vi "BallChaseAuton.vi"(9 "milliseconds to fire":u32=750) -> ()   [LabVIEW 2013]
uses:
  Auton sequence.ctl
  Events.vi
  TwoBallAuton.ctl
panel:
  out "State":T1=enum."GetBall"
  out "GrabCount":i32
  out "Direction saw last":dbl
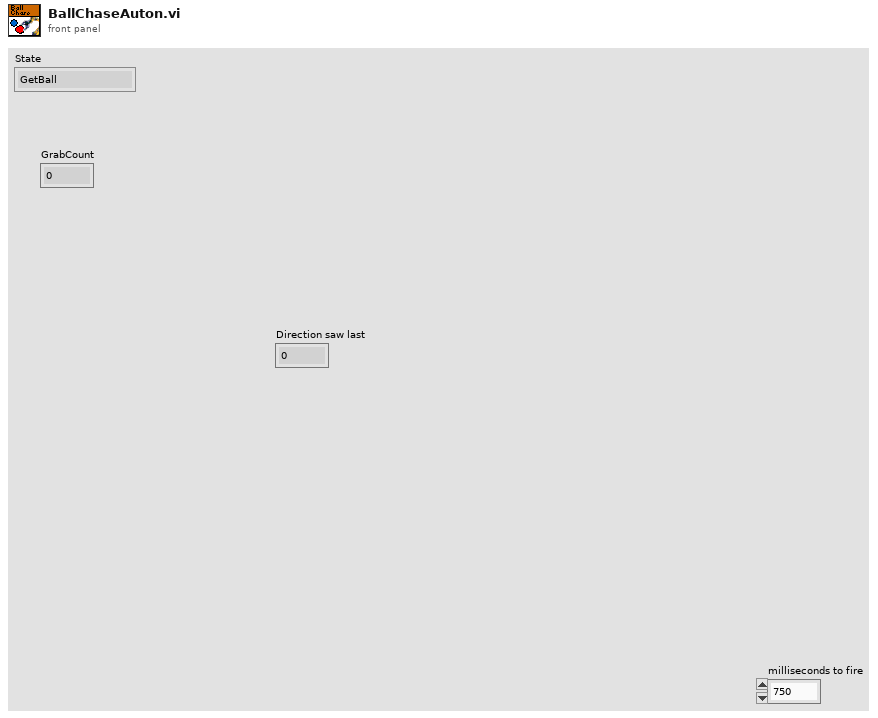
[diagram p1: front panel]
types:
  T1 = typedef "TwoBallAuton.ctl" = enum16{"Start", "LineUp", "Fire", "Reload", "GetBall", "Finish"}
  T2 = typedef "Auton sequence.ctl" = enum16{"Done", "move", "Shoot Ball 2", "Aquire target", "Ball chase", "Turn 90 ", "Shoot Ball 1"}
  T3 = typedef "WPI_SolenoidValue.ctl" = enum16{"Off", "On", "Forward", "Reverse"}
  T4 = cluster{"Ultrasonic Distance (In)":dbl, "Gyro":dbl, "TopAquisition sensor":bool, "Encoder distance":dbl, "Encoder rate":dbl, "Encoder direction":bool, "winch engaged?":T3, "Motor Values":dbl[], "Latch encoder":u32, "BottomAquistion":bool, "BottomAquistion 2":bool}
  T5 = cluster{"Translate":dbl, "Y-Axis (Backward Speed)":dbl, "Rotate":dbl, "Tank right side":dbl, "axis 5":dbl, "axis 6":dbl, "Use gyro":bool, "Exponential\ndrive":bool, "Ring light":bool}
  T6 = cluster{"Reloading?":bool, "Throw":bool, "Ready?":bool, "Truss throw":bool, "Power is high?":bool, "Automatic relaod?":bool, "Manuall servo":bool}
  T7 = typedef "Eventgrab.ctl" = cluster{"Grab":bool, "GroundPass":bool, "Test Aqaure":dbl, "Shoulder up or down?":bool}
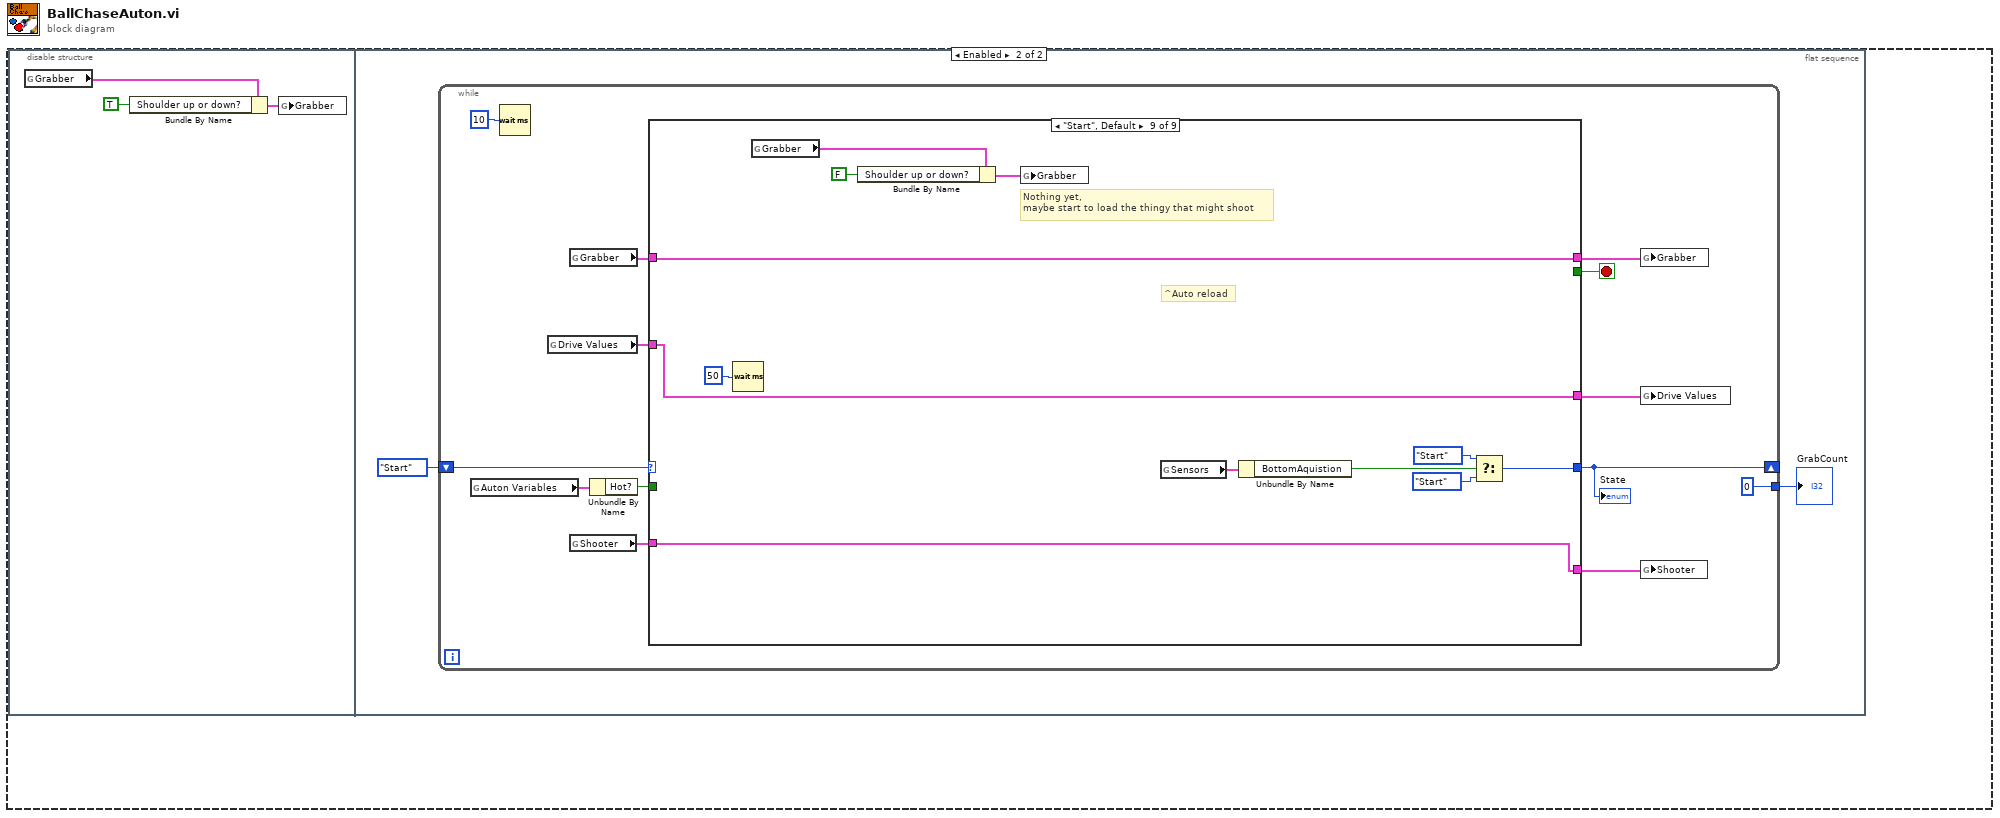
[diagram p0: block diagram]
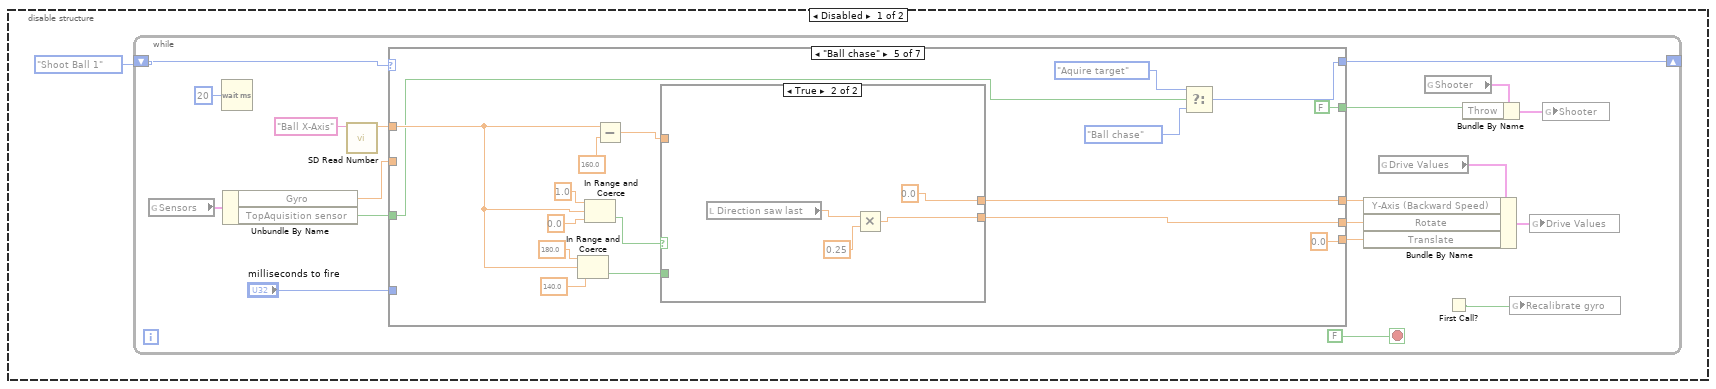
[diagram p2: hidden frame]
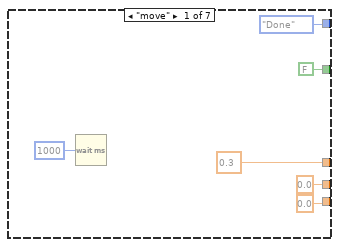
[diagram p3: hidden frame]
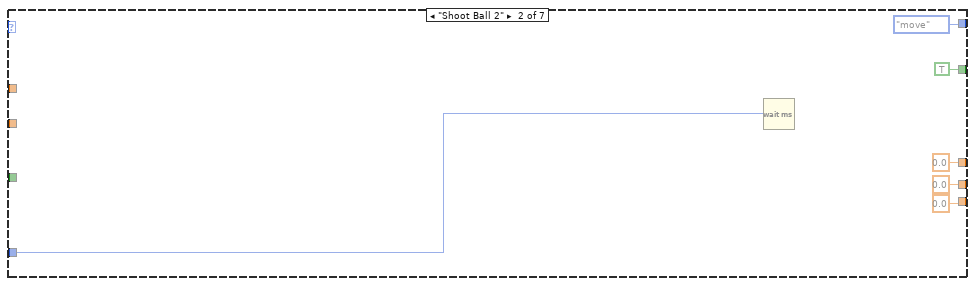
[diagram p4: hidden frame]
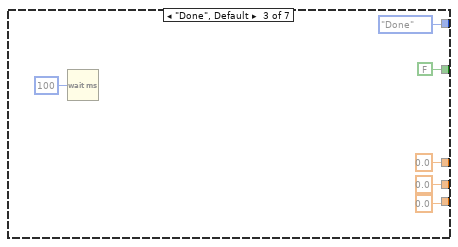
[diagram p5: hidden frame]
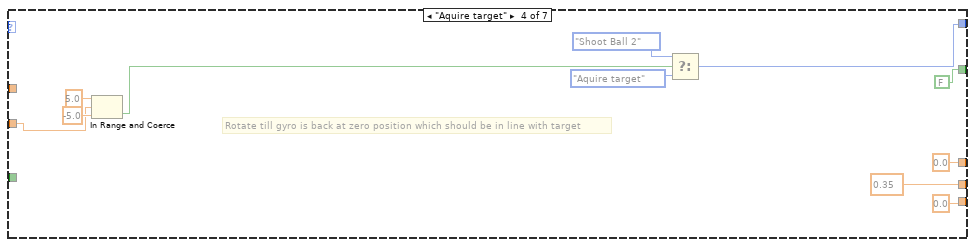
[diagram p6: hidden frame]
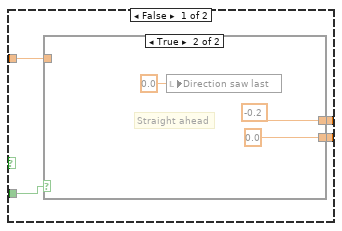
[diagram p7: hidden frame]
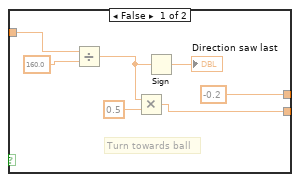
[diagram p8: hidden frame]
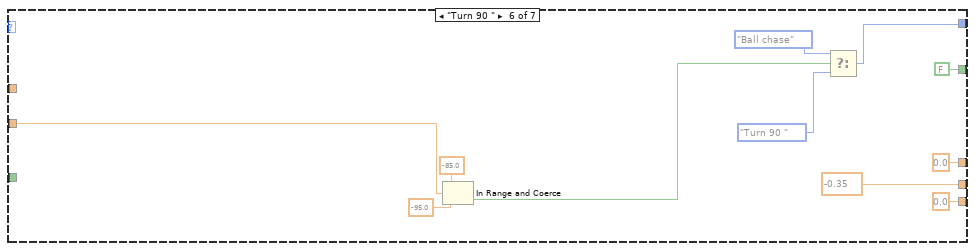
[diagram p9: hidden frame]
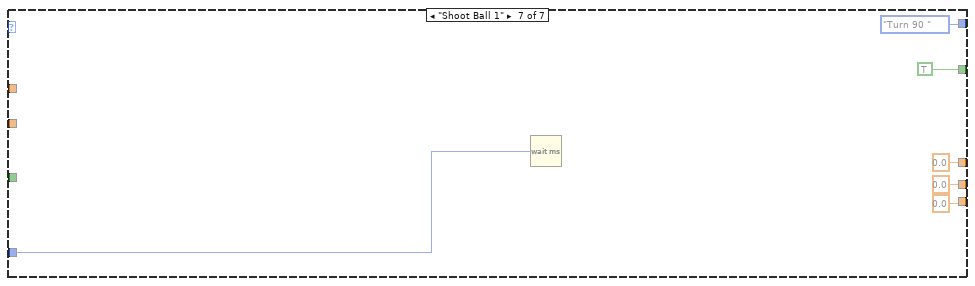
[diagram p10: hidden frame]
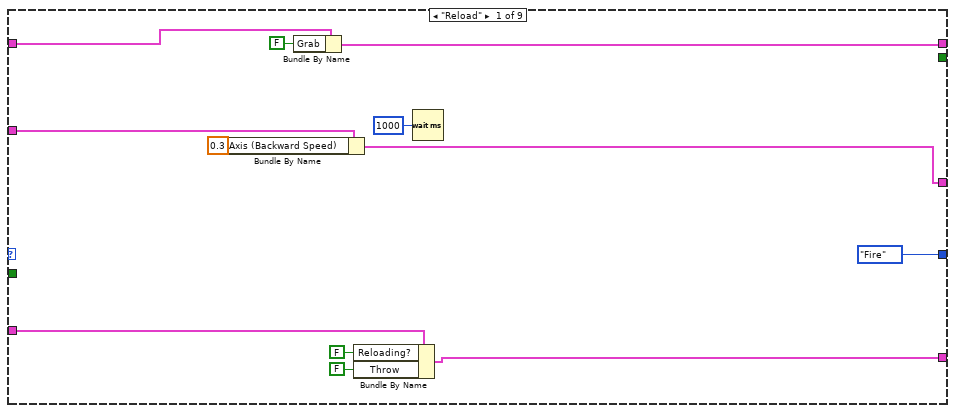
[diagram p11: hidden frame]
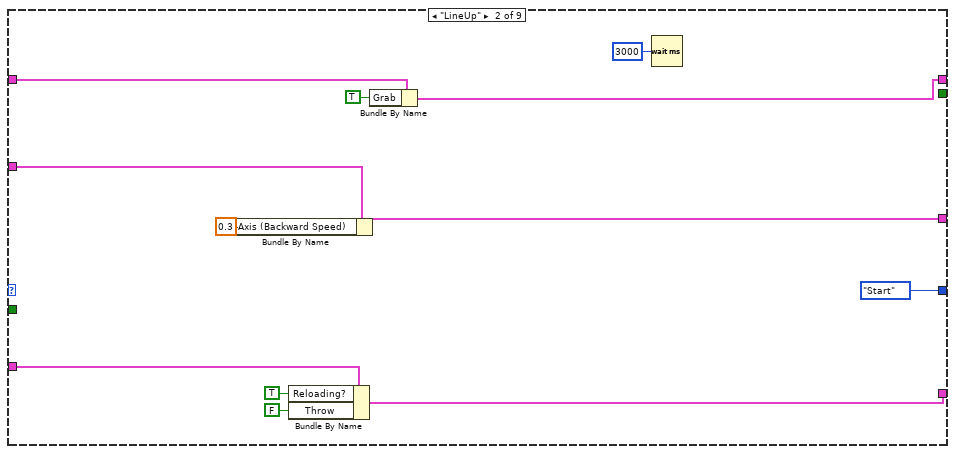
[diagram p12: hidden frame]
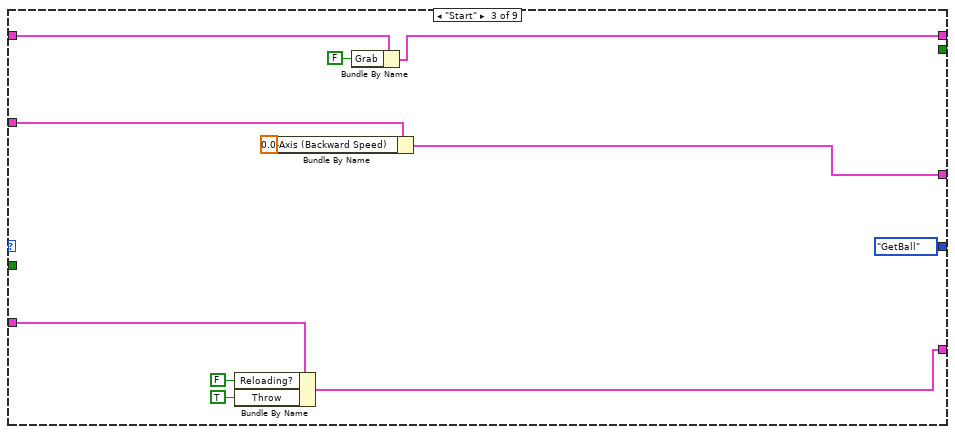
[diagram p13: hidden frame]
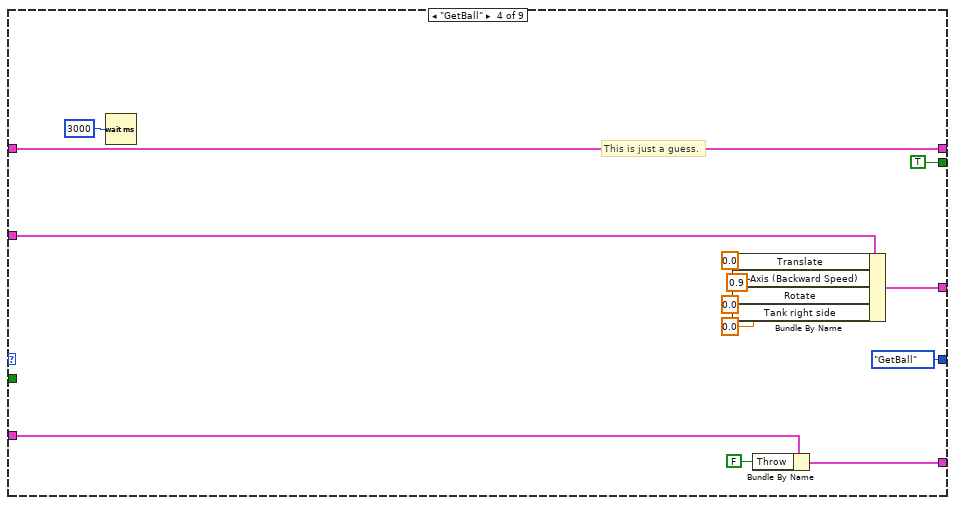
[diagram p14: hidden frame]
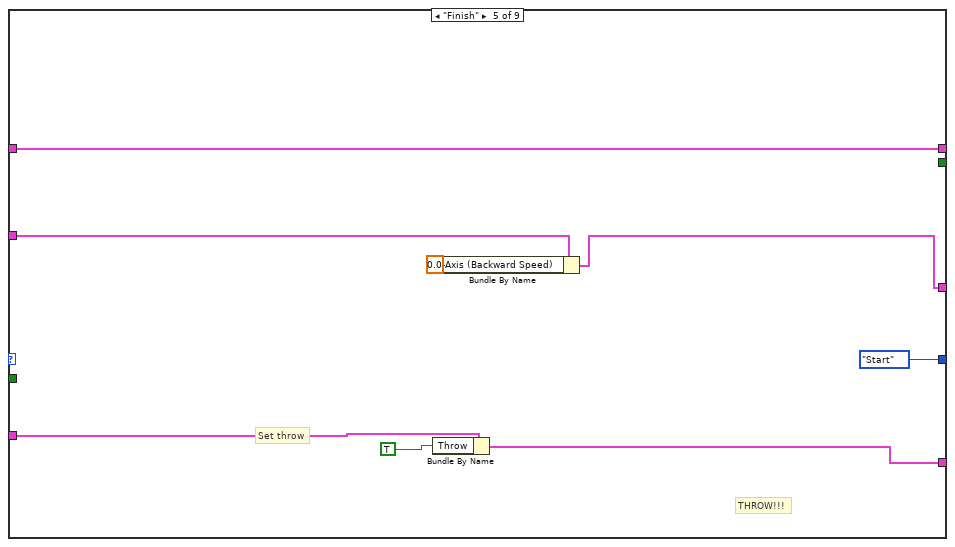
[diagram p15: hidden frame]
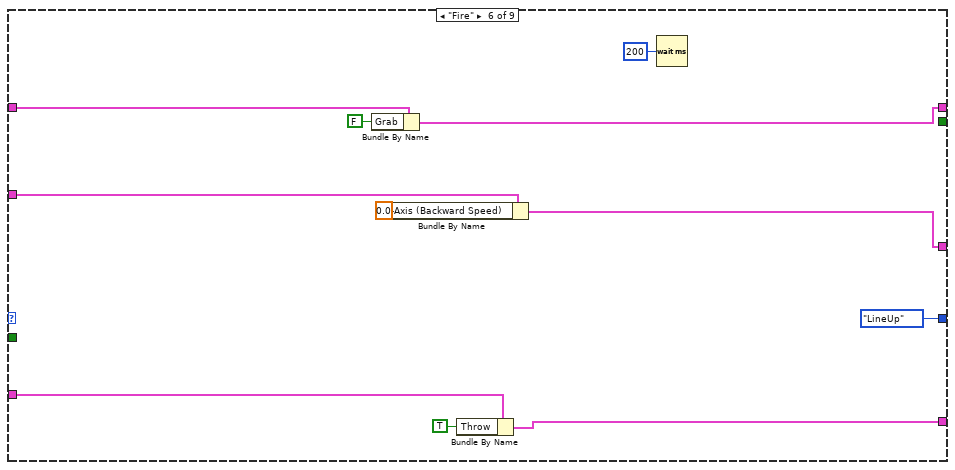
[diagram p16: hidden frame]
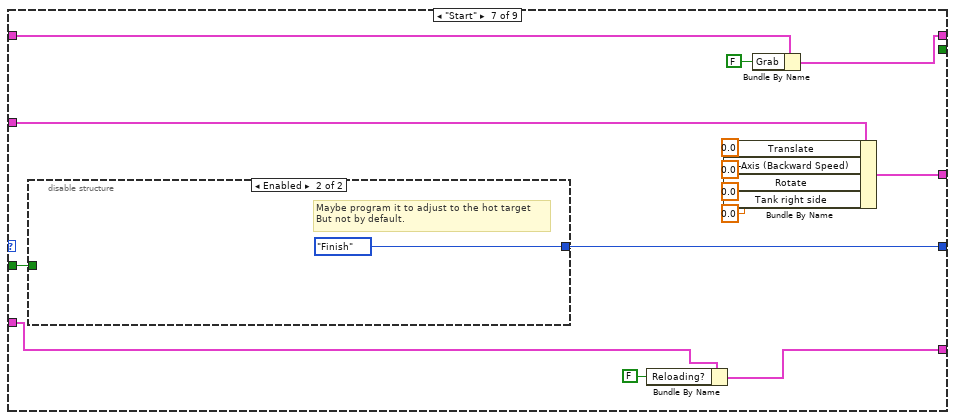
[diagram p17: hidden frame]
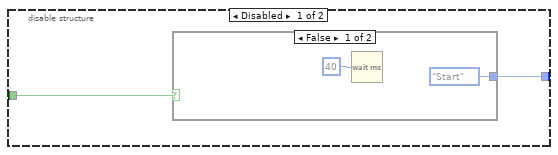
[diagram p18: hidden frame]
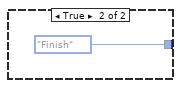
[diagram p19: hidden frame]
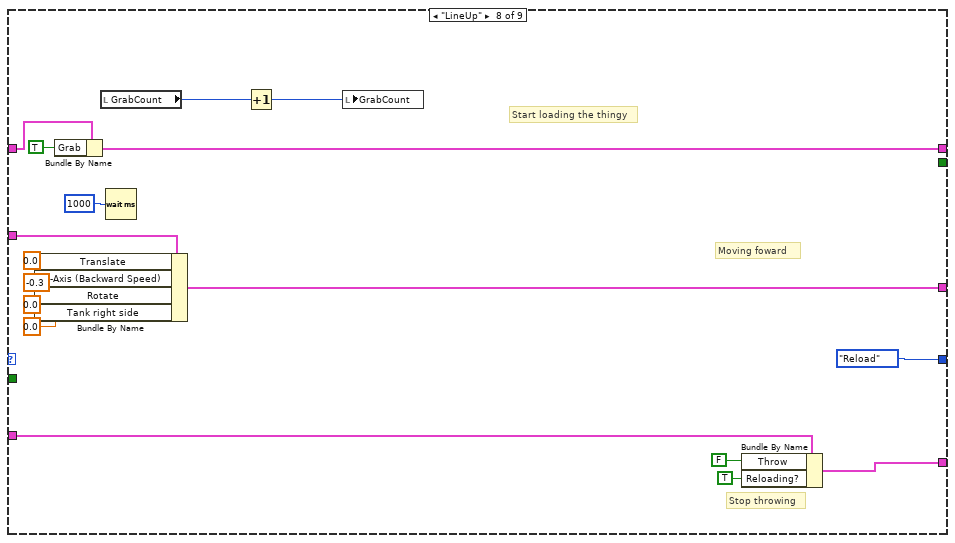
[diagram p20: hidden frame]
diagram:
  n1 = disable-structure shown="Enabled" {
    frame Disabled {
      n2 = while {
        shift-right: [w12] -> _
        shift-left: Auton_sequence."Shoot Ball 1" -> [w19]
        stop <- FALSE stop-if-true
        n3 = global read "Events.vi" "Sensors"() -> (w3:T4)
        n4 = Wait (ms)(milliseconds to wait=u32 20) -> ()  [unwired: 1 out]
        n5 = Unbundle By Name(w3) -> ("Gyro"=w10:dbl, "TopAquisition sensor"=w9:bool)
        n6 = call <vilib>:"SD Read Number.vi"("Name"="Ball X-Axis") -> ("Numeric"=w16:dbl)  [unwired: 8 in, 2 out]
        n7 = case shown="\"Ball chase\"" w19 {
          tunnel: w16 -> [_ _ _ _ w58 _ _]
          tunnel: [0.3 ("Forward Speed") 0.0 ("Forward Speed") 0.0 ("Forward Speed") 0.0 ("Forward Speed") w57 0.0 ("Forward Speed") 0.0 ("Forward Speed")] -> w15
          tunnel: [0.0 ("Rotate") 0.0 ("Rotate") 0.0 ("Rotate") 0.35 ("Rotate") w56 -0.35 ("Rotate") 0.0 ("Rotate")] -> w13
          tunnel: [0.0 ("Translate") 0.0 ("Translate") 0.0 ("Translate") 0.0 ("Translate") 0.0 ("Translate") 0.0 ("Translate") 0.0 ("Translate")] -> w14
          tunnel: [Auton_sequence."Done" Auton_sequence."move" Auton_sequence."Done" w47 w53 w89 Auton_sequence."Turn 90 "] -> w12
          tunnel: [FALSE TRUE FALSE FALSE FALSE FALSE TRUE] -> w11
          tunnel: w10 -> [_ _ _ w39 _ w85 _]
          tunnel: w9 -> [_ _ _ _ w50 _ _]
          tunnel: "milliseconds to fire" -> [_ w27 _ _ _ _ w96]
          frame "move" {
            n8 = Wait (ms)(milliseconds to wait=u32 1000) -> ()  [unwired: 1 out]
          }
          frame "Shoot Ball 2" {
            n9 = Wait (ms)(milliseconds to wait=w27) -> ()  [unwired: 1 out]
          }
          frame "Done", Default {
            n10 = Wait (ms)(milliseconds to wait=u32 100) -> ()  [unwired: 1 out]
          }
          frame "Aquire target" {
            # "Rotate till gyro is back at zero position which should be in line with target"
            n11 = In Range and Coerce(upper limit=5.0, x=w39, lower limit=-5.0) -> (In Range?=w46:bool)  [unwired: 1 out]
            n12 = Select(t=Auton_sequence."Shoot Ball 2", s=w46, f=Auton_sequence."Aquire target") -> (s? t:f=w47:T2)
          }
          frame "Ball chase" {
            n13 = In Range and Coerce(upper limit=180.0, x=w58, lower limit=140.0) -> (In Range?=w59:bool)  [unwired: 1 out]
            n14 = In Range and Coerce(upper limit=1.0, x=w58, lower limit=0.0) -> (In Range?=w60:bool)  [unwired: 1 out]
            n15 = Subtract(x=w58, y=160.0) -> (x-y=w65:dbl)
            n16 = case shown="True" w60 {
              tunnel: w65 -> [w69 _]
              tunnel: w59 -> [w70 _]
              tunnel: [w68 w82] -> w56
              tunnel: [w67 0.0 ("Forward Speed")] -> w57
              frame False {
                n17 = case shown="True" w70 {
                  tunnel: w69 -> [w77 _]
                  tunnel: [w74 0.0] -> w68
                  tunnel: [-0.2 -0.2] -> w67
                  frame False {
                    # "Turn towards ball"
                    n18 = Divide(x=w77, y=160.0) -> (x/y=w72:dbl)
                    n19 = Multiply(x=w72, y=0.5) -> (x*y=w74:dbl)
                    n20 = Sign(1:w72) -> (0:→"Direction saw last":dbl)
                  }
                  frame True {
                    # "Straight ahead"
                    n21 = local write "Direction saw last"(0.0 ("Direction saw last")) -> ()
                  }
                }
              }
              frame True {
                n22 = local read "Direction saw last"() -> (w81:dbl)
                n23 = Multiply(x=w81, y=0.25) -> (x*y=w82:dbl)
              }
            }
            n24 = Select(t=Auton_sequence."Aquire target", s=w50, f=Auton_sequence."Ball chase") -> (s? t:f=w53:T2)
          }
          frame "Turn 90 " {
            n25 = In Range and Coerce(upper limit=-85.0, x=w85, lower limit=-95.0) -> (In Range?=w87:bool)  [unwired: 1 out]
            n26 = Select(t=Auton_sequence."Ball chase", s=w87, f=Auton_sequence."Turn 90 ") -> (s? t:f=w89:T2)
          }
          frame "Shoot Ball 1" {
            n27 = Wait (ms)(milliseconds to wait=w96) -> ()  [unwired: 1 out]
          }
        }
        n28 = global read "Events.vi" "Drive Values"() -> (w5:T5)
        n29 = Bundle By Name(cluster=w5, "Y-Axis (Backward Speed)"=w15, "Rotate"=w13, "Translate"=w14) -> (w7:T5)
        n30 = global read "Events.vi" "Shooter"() -> (w4:T6)
        n31 = First Call?() -> (First Call?: T/F=w8:bool)
        n32 = Bundle By Name(cluster=w4, "Throw"=w11) -> (w6:T6)
        n33 = global write "Events.vi" "Recalibrate gyro"(w8) -> ()
        n34 = global write "Events.vi" "Drive Values"(w7) -> ()
        n35 = global write "Events.vi" "Shooter"(w6) -> ()
      }
    }
    frame Enabled {
      n36 = flat-sequence {
        frame #0 {
          n37 = global read "Events.vi" "Grabber"() -> (w103:T7)
          n38 = Bundle By Name(cluster=w103, "Shoulder up or down?"=TRUE) -> (w104:T7)
          n39 = global write "Events.vi" "Grabber"(w104) -> ()
        }
        frame #1 {
          n40 = while {
            shift-right: [w118] -> _
            shift-left: TwoBallAuton."Start" -> [w107]
            tunnel: [0] -> w105
            stop <- w108 stop-if-true
            n41 = global read "Events.vi" "Auton Variables"() -> (w113:cluster{"Hot?":bool, "WhichAuton":string})
            n42 = Wait (ms)(milliseconds to wait=u32 10) -> ()  [unwired: 1 out]
            n43 = global read "Events.vi" "Drive Values"() -> (w115:T5)
            n44 = global read "Events.vi" "Grabber"() -> (w114:T7)
            n45 = global read "Events.vi" "Shooter"() -> (w116:T6)
            n46 = Unbundle By Name(w113) -> ("Hot?"=w112:bool)
            n47 = case shown="\"Start\", Default" w107 {
              tunnel: [TwoBallAuton."Fire" TwoBallAuton."Start" TwoBallAuton."GetBall" TwoBallAuton."GetBall" TwoBallAuton."Start" TwoBallAuton."LineUp" w190 TwoBallAuton."Reload" w231] -> w118
              tunnel: [_ _ _ TRUE _ _ _ _ _] -> w108
              tunnel: w112 -> [_ _ _ _ _ _ w191 _ _]
              tunnel: w116 -> [w124 w137 w148 w157 w173 w186 w189 w211 w233]
              tunnel: w115 -> [w131 w143 w151 w160 w171 w183 w196 w220 w235]
              tunnel: w114 -> [w127 w140 w154 w165 w175 w180 w194 w213 w234]
              tunnel: [w130 w142 w150 w159 w170 w182 w195 w215 w235] -> w111
              tunnel: [w126 w139 w153 w165 w175 w179 w192 w214 w234] -> w110
              tunnel: [w123 w136 w147 w156 w172 w185 w188 w210 w233] -> w109
              frame "Reload" {
                n48 = Bundle By Name(cluster=w131, "Y-Axis (Backward Speed)"=0.3 ("Forward Speed")) -> (w130:T5)
                n49 = Bundle By Name(cluster=w127, "Grab"=FALSE) -> (w126:T7)
                n50 = Bundle By Name(cluster=w124, "Reloading?"=FALSE, "Throw"=FALSE) -> (w123:T6)
                n51 = Wait (ms)(milliseconds to wait=u32 1000) -> ()  [unwired: 1 out]
              }
              frame "LineUp" {
                n52 = Bundle By Name(cluster=w143, "Y-Axis (Backward Speed)"=0.3 ("Forward Speed")) -> (w142:T5)
                n53 = Bundle By Name(cluster=w137, "Reloading?"=TRUE, "Throw"=FALSE) -> (w136:T6)
                n54 = Bundle By Name(cluster=w140, "Grab"=TRUE) -> (w139:T7)
                n55 = Wait (ms)(milliseconds to wait=u32 3000) -> ()  [unwired: 1 out]
              }
              frame "Start" {
                n56 = Bundle By Name(cluster=w148, "Reloading?"=FALSE, "Throw"=TRUE) -> (w147:T6)
                n57 = Bundle By Name(cluster=w151, "Y-Axis (Backward Speed)"=0.0 ("Forward Speed")) -> (w150:T5)
                n58 = Bundle By Name(cluster=w154, "Grab"=FALSE) -> (w153:T7)
              }
              frame "GetBall" {
                # "This is just a guess."
                n59 = Wait (ms)(milliseconds to wait=u32 3000) -> ()  [unwired: 1 out]
                n60 = Bundle By Name(cluster=w160, "Translate"=0.0, "Y-Axis (Backward Speed)"=0.9 ("Forward Speed"), "Rotate"=0.0, "Tank right side"=0.0) -> (w159:T5)
                n61 = Bundle By Name(cluster=w157, "Throw"=FALSE) -> (w156:T6)
              }
              frame "Finish" {
                # "Set throw"
                # "THROW!!!"
                n62 = Bundle By Name(cluster=w171, "Y-Axis (Backward Speed)"=0.0 ("Forward Speed")) -> (w170:T5)
                n63 = Bundle By Name(cluster=w173, "Throw"=TRUE) -> (w172:T6)
              }
              frame "Fire" {
                n64 = Bundle By Name(cluster=w180, "Grab"=FALSE) -> (w179:T7)
                n65 = Bundle By Name(cluster=w183, "Y-Axis (Backward Speed)"=0.0 ("Forward Speed")) -> (w182:T5)
                n66 = Bundle By Name(cluster=w186, "Throw"=TRUE) -> (w185:T6)
                n67 = Wait (ms)(milliseconds to wait=u32 200) -> ()  [unwired: 1 out]
              }
              frame "Start" {
                n68 = disable-structure shown="Enabled" {
                  disable-tunnel: w191 -> [w202 _]
                  disable-tunnel: [w201 TwoBallAuton."Finish"] -> w190
                  frame Disabled {
                    n69 = case shown="False" w202 {
                      tunnel: [TwoBallAuton."Start" TwoBallAuton."Finish"] -> w201
                      frame False {
                        n70 = Wait (ms)(milliseconds to wait=u32 40) -> ()  [unwired: 1 out]
                      }
                      frame True {
                      }
                    }
                  }
                  frame Enabled {
                    # "Maybe program it to adjust to the hot target\nBut not by default."
                  }
                }
                n71 = Bundle By Name(cluster=w189, "Reloading?"=FALSE) -> (w188:T6)
                n72 = Bundle By Name(cluster=w196, "Translate"=0.0, "Y-Axis (Backward Speed)"=0.0 ("Forward Speed"), "Rotate"=0.0, "Tank right side"=0.0) -> (w195:T5)
                n73 = Bundle By Name(cluster=w194, "Grab"=FALSE) -> (w192:T7)
              }
              frame "LineUp" {
                # "Stop throwing"
                # "Moving foward"
                # "Start loading the thingy"
                n74 = Bundle By Name(cluster=w220, "Translate"=0.0, "Y-Axis (Backward Speed)"=-0.3 ("Forward Speed"), "Rotate"=0.0, "Tank right side"=0.0) -> (w215:T5)
                n75 = Bundle By Name(cluster=w213, "Grab"=TRUE) -> (w214:T7)
                n76 = local read "GrabCount"() -> (w223:i32)
                n77 = Wait (ms)(milliseconds to wait=u32 1000) -> ()  [unwired: 1 out]
                n78 = Increment(x=w223) -> (x+1=w222:i32)
                n79 = local write "GrabCount"(w222) -> ()
                n80 = Bundle By Name(cluster=w211, "Throw"=FALSE, "Reloading?"=TRUE) -> (w210:T6)
              }
              frame "Start", Default {
                # "^Auto reload"
                # "Nothing yet,\nmaybe start to load the thingy that might shoot"
                n81 = Wait (ms)(milliseconds to wait=u32 50) -> ()  [unwired: 1 out]
                n82 = global read "Events.vi" "Grabber"() -> (w225:T7)
                n83 = Bundle By Name(cluster=w225, "Shoulder up or down?"=FALSE) -> (w226:T7)
                n84 = global write "Events.vi" "Grabber"(w226) -> ()
                n85 = global read "Events.vi" "Sensors"() -> (w232:T4)
                n86 = Unbundle By Name(w232) -> ("BottomAquistion"=w230:bool)
                n87 = Select(t=TwoBallAuton."Start", s=w230, f=TwoBallAuton."Start") -> (s? t:f=w231:T1)
              }
            }
            "State" <- w118
            n88 = global write "Events.vi" "Grabber"(w110) -> ()
            n89 = global write "Events.vi" "Drive Values"(w111) -> ()
            n90 = global write "Events.vi" "Shooter"(w109) -> ()
          }
          "GrabCount" <- w105
        }
      }
    }
  }
